vi "crio_FPGA_PWM_efficient.vi"() -> ()   [LabVIEW 2019]
uses:
  <vilib>/rvi/Analysis/control/PID/Typedef/niFpgaPID_PIGains.ctl
  <vilib>/rvi/Analysis/control/PID/Typedef/niFpgaPID_ManualControl.ctl
  <vilib>/rvi/Analysis/control/PID/Typedef/niFpgaPID_OutputRange.ctl
  <vilib>/rvi/Emulation/niFpgaSctlEmulationGetInTimedLoop.vi
  <vilib>/rvi/Emulation/niFpgaProcessEmulError.vi
  <vilib>/rvi/eio/common/nirviEmuTemplateMethod_errors.vi
  <vilib>/rvi/Emulation/niFpgaGetClockAttributes.vi
  <vilib>/rvi/Emulation/niFpgaEmulationReportErrorSimple.vi
  <vilib>/rvi/Emulation/niFpgaCriticalErrorInLSC.vi
  <vilib>/rvi/Analysis/control/PID/SubVIs/niFpgaPID_PIWrapper.vi
  <vilib>/eio/EIOMethodNode/EIOMethodNode.xnode
  <vilib>/eio/EIONode/EIONode.xnode
panel:
  out "ControllerPWM Output":sgl
  in  "manual control":T1 {"manual input (0)" scale=-1.0..1.0}
  in  "setpoint":i32
  in  "gains":T2 {"proportional gain" step=0.125}
  in  "Debug: ConnectorA/DIO15":bool
  in  "Debug: ConnectorA/DIO14":bool
  in  "Encoder Debug":bool
  in  "Loop Timer DAQ":u32=1 caption="Loop Time(uSec)"
  in  "Position Reset":bool
  out "Position (Counts)":i64
  out "B":bool
  out "A":bool
  out "B'":bool
  out "A'":bool
  in  "Velocity Interval (uSec)":u32=1000
  out "Acceleration (Counts/Interval)":i32
  out "Velocity (Counts/Interval)":i32
  in  "stop":bool
  in  "DC PWM Period (microsec)":i16=50
  # "DRV8256 Specs:\n\n0 0: Brake Low\n1 1: Brake High\nPWM 0\n0 PWM"
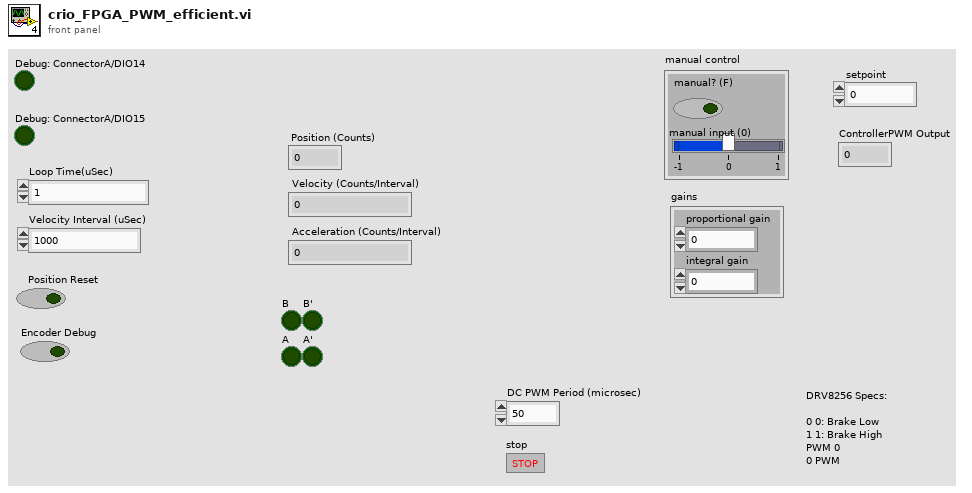
[diagram p1: front panel]
types:
  T1 = typedef "niFpgaPID_ManualControl.ctl" = cluster{"manual? (F)":bool, "manual input (0)":sgl}
  T2 = typedef "niFpgaPID_PIGains.ctl" = cluster{"proportional gain":sgl, "integral gain":sgl}
  T3 = typedef "niFpgaPID_OutputRange.ctl" = cluster{"output high (Inf)":sgl, "output low (-Inf)":sgl}
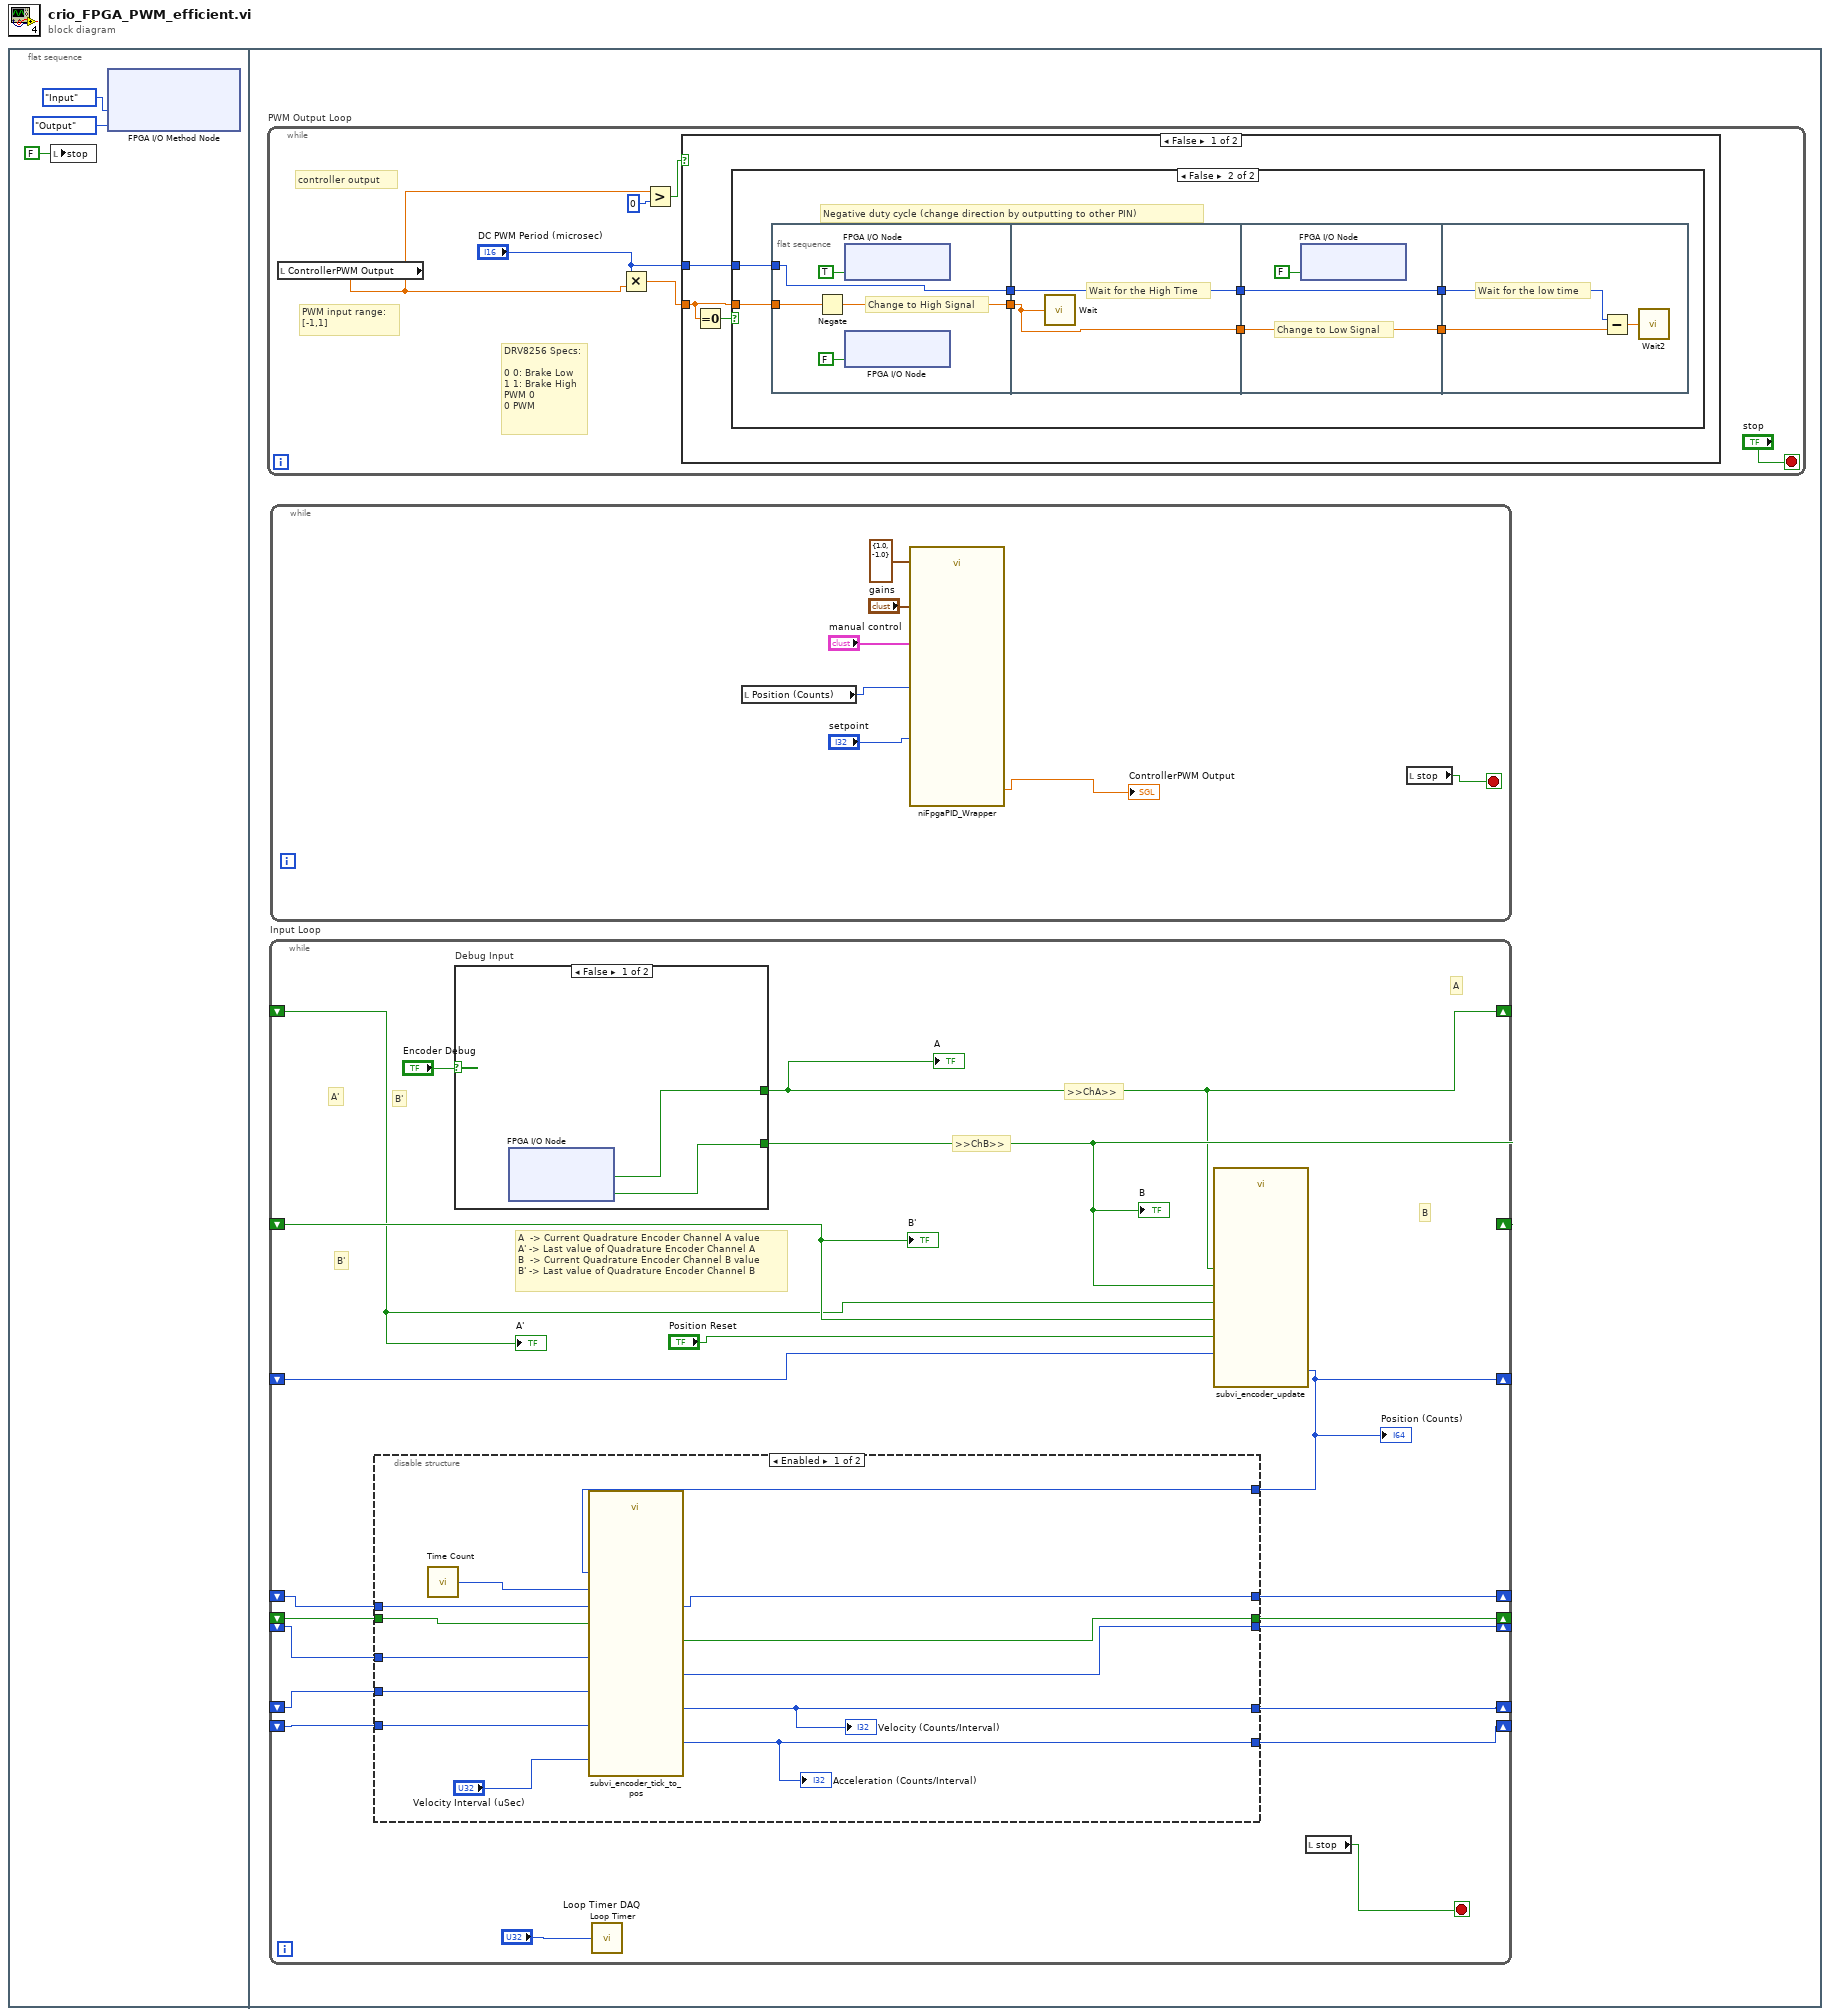
[diagram p0: block diagram]
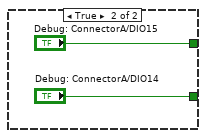
[diagram p3: hidden frame]
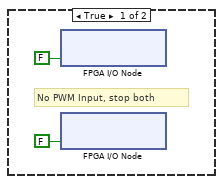
[diagram p4: hidden frame]
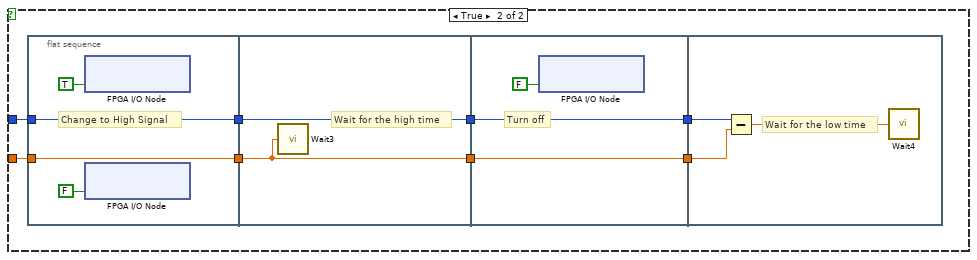
[diagram p5: hidden frame]
diagram:
  n1 = flat-sequence {
    frame #0 {
      n2 = local write "stop"(FALSE ("stop")) -> ()
      n3 = xnode "FPGA I/O Method Node"("DIO 7:4"=enum8{"No Change", "Input", "Output"}."Input", "DIO 3:0"=enum8{"No Change", "Input", "Output"}."Output") -> ()  [unwired: 1 in, 1 out]
    }
    frame #1 {
      n4 = while "PWM Output Loop" {
        stop <- "stop" stop-if-true
        # "PWM input range:\n[-1,1]"
        # "DRV8256 Specs:\n\n0 0: Brake Low\n1 1: Brake High\nPWM 0\n0 PWM"
        # "controller output"
        n5 = local read "ControllerPWM Output"() -> (w48:sgl)
        n6 = Multiply(x="DC PWM Period (microsec)", y=w48) -> (x*y=w50:sgl)
        n7 = Greater?(x=w48, y=i16 0) -> (0:w51:bool)
        n8 = case shown="False" w51 {
          tunnel: w50 -> [w56 w87]
          tunnel: "DC PWM Period (microsec)" -> [w54 w86]
          frame False {
            n9 = Equal To 0?(x=w56) -> (x = 0?=w55:bool)
            n10 = case shown="False" w55 {
              tunnel: w56 -> [_ w66]
              tunnel: w54 -> [_ w59]
              frame True {
                # "No PWM Input, stop both"
                n11 = xnode "FPGA I/O Node"("Mod1/DIO1"=FALSE) -> ()  [unwired: 1 in, 1 out]
                n12 = xnode "FPGA I/O Node"("Mod1/DIO0"=FALSE) -> ()  [unwired: 1 in, 1 out]
              }
              frame False {
                # "Negative duty cycle (change direction by outputting to other PIN)"
                n13 = flat-sequence {
                  tunnel: w66 -> [w69]
                  tunnel: [w68] -> w65
                  tunnel: [w67] -> w60
                  tunnel: w59 -> [w67]
                  tunnel: w65 -> [w73]
                  tunnel: [w73] -> w64
                  tunnel: [w72] -> w61
                  tunnel: w60 -> [w72]
                  tunnel: w64 -> [w75]
                  tunnel: [w75] -> w63
                  tunnel: [w74] -> w62
                  tunnel: w61 -> [w74]
                  tunnel: w63 -> [w79]
                  tunnel: w62 -> [w78]
                  frame #0 {
                    # "Change to High Signal"
                    n14 = Negate(x=w69) -> (-x=w68:sgl)
                    n15 = xnode "FPGA I/O Node"("Mod1/DIO1"=TRUE) -> ()  [unwired: 1 in, 1 out]
                    n16 = xnode "FPGA I/O Node"("Mod1/DIO0"=FALSE) -> ()  [unwired: 1 in, 1 out]
                  }
                  frame #1 {
                    # "Wait for the High Time"
                    n17 = call "Wait"("Count(uSec)"=w73) -> ()  [unwired: 1 out]
                  }
                  frame #2 {
                    # "Change to Low Signal"
                    n18 = xnode "FPGA I/O Node"("Mod1/DIO1"=FALSE) -> ()  [unwired: 1 in, 1 out]
                  }
                  frame #3 {
                    # "Wait for the low time"
                    n19 = Subtract(x=w78, y=w79) -> (x-y=w77:sgl)
                    n20 = call "Wait2"("Count(uSec)"=w77) -> ()  [unwired: 1 out]
                  }
                }
              }
            }
          }
          frame True {
            n21 = flat-sequence {
              tunnel: w87 -> [w88]
              tunnel: w86 -> [w89]
              tunnel: [w89] -> w83
              tunnel: [w88] -> w82
              tunnel: [w93] -> w84
              tunnel: w83 -> [w93]
              tunnel: w82 -> [w92]
              tunnel: [w92] -> w81
              tunnel: [w95] -> w85
              tunnel: w84 -> [w95]
              tunnel: w81 -> [w94]
              tunnel: [w94] -> w80
              tunnel: w85 -> [w99]
              tunnel: w80 -> [w97]
              frame #0 {
                # "Change to High Signal"
                n22 = xnode "FPGA I/O Node"("Mod1/DIO0"=TRUE) -> ()  [unwired: 1 in, 1 out]
                n23 = xnode "FPGA I/O Node"("Mod1/DIO1"=FALSE ("ConnectorB/DIO9")) -> ()  [unwired: 1 in, 1 out]
              }
              frame #1 {
                # "Wait for the high time"
                n24 = call "Wait3"("Count(uSec)"=w92) -> ()  [unwired: 1 out]
              }
              frame #2 {
                # "Turn off"
                n25 = xnode "FPGA I/O Node"("Mod1/DIO0"=FALSE) -> ()  [unwired: 1 in, 1 out]
              }
              frame #3 {
                # "Wait for the low time"
                n26 = Subtract(x=w99, y=w97) -> (x-y=w98:sgl)
                n27 = call "Wait4"("Count(uSec)"=w98) -> ()  [unwired: 1 out]
              }
            }
          }
        }
      }
      n28 = while "Input Loop" {
        shift-right: [w24] -> _
        shift-left: _ -> [w27]
        shift-right: [w23] -> _
        shift-left: _ -> [w26]
        shift-right: [w19] -> _
        shift-left: _ -> [w25]
        shift-right: [w12] -> _
        shift-left: _ -> [w22]
        shift-right: [w13] -> _
        shift-left: _ -> [w21]
        shift-right: [w20] -> _
        shift-left: _ -> [w18]
        shift-right: [w17] -> _
        shift-left: _ -> [w16]
        shift-right: [w15] -> _
        shift-left: _ -> [w14]
        stop <- w11 stop-if-true
        # "B'"
        # ">>ChB>>"
        # ">>ChA>>"
        # "A'"
        # "A  -> Current Quadrature Encoder Channel A value\nA' -> Last value of Quadrature Encoder Channel A\nB  -> Current Quadrature Encoder Channel B value\nB' -> Last value of Quadrature Encoder Channel B"
        # "B'"
        # "B"
        # "A"
        n29 = case "Debug Input" shown="False" "Encoder Debug" {
          tunnel: [w45 "Debug: ConnectorA/DIO15"] -> w23
          tunnel: [w44 "Debug: ConnectorA/DIO14"] -> w24
          frame False {
            n30 = xnode "FPGA I/O Node"() -> ("Mod1/DIO4"=w45:bool, "Mod1/DIO5"=w44:bool)  [unwired: 2 in, 2 out]
          }
          frame True {
          }
        }
        "B" <- w24
        "A" <- w23
        n31 = call "Loop Timer"("Count(uSec)"="Loop Timer DAQ") -> ()  [unwired: 1 out]
        n32 = call "subvi_encoder_update.vi"("Position Reset"="Position Reset", "Tick'"=w25, "A"=w23, "B'"=w27, "A'"=w26, "B"=w24) -> ("Tick"=w19:i32)  [unwired: 5 in]
        "Position (Counts)" <- w19
        n33 = disable-structure shown="Enabled" {
          disable-tunnel: w22 -> [w42 _]
          disable-tunnel: w21 -> [w41 _]
          disable-tunnel: [w40 _] -> w20
          disable-tunnel: w19 -> [w39 _]
          disable-tunnel: w18 -> [w38 _]
          disable-tunnel: [w37 _] -> w17
          disable-tunnel: w16 -> [w36 _]
          disable-tunnel: [w35 _] -> w15
          disable-tunnel: w14 -> [w34 _]
          disable-tunnel: [w32 _] -> w13
          disable-tunnel: [w31 _] -> w12
          frame Enabled {
            n34 = call "Time Count"() -> ("Tick Count(uSec)"=w33:u32)
            n35 = call "subvi_encoder_tick_to_pos.vi"("Velocity Interval (uSec)"="Velocity Interval (uSec)", "Raw Tick"=w39, "Waited?'"=w36, "Tick Count(uSec)'"=w34, "p'"=w38, "Time Count"=w33, "a'"=w41, "v'"=w42) -> ("Waited?"=w37:bool, "Tick Count(uSec)"=w35:u32, "p"=w40:i32, "a"=w32:i32, "v"=w31:i32)  [unwired: 3 in]
            "Acceleration (Counts/Interval)" <- w32
            "Velocity (Counts/Interval)" <- w31
          }
          frame Disabled {
          }
        }
        n36 = local read "stop"() -> (w11:bool)
        "B'" <- w27
        "A'" <- w26
      }
      n37 = while {
        stop <- w10 stop-if-true
        n38 = local read "Position (Counts)"() -> (w9:i64)
        n39 = call-poly <vilib>:"niFpgaPID_Wrapper.vi"("setpoint"="setpoint", "process variable"=w9, "manual control"="manual control", "gains"="gains", "output range"=T3 {"output high (Inf)"=1.0, "output low (-Inf)"=-1.0}) -> ("output"=→"ControllerPWM Output":sgl)  [unwired: 8 in, 2 out]
        n40 = local read "stop"() -> (w10:bool)
      }
    }
  }
